vi "DISP err unknow request.vi"(11 "String":string) -> ()   [LabVIEW 2020]
uses:
  MsgBox.vi
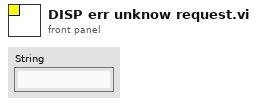
[diagram p1: front panel]
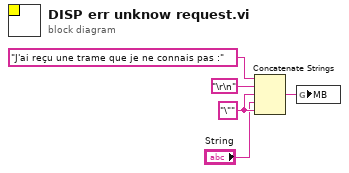
[diagram p0: block diagram]
diagram:
  w3 = "\"" ("chaîne")
  n1 = Concatenate Strings("J'ai reçu une trame que je ne connais pas :" ("MSG"), "\r\n", w3, "String", w3) -> (w5:string)
  n2 = global write "MsgBox.vi" "MB"(w5) -> ()
